vi "Capture the Project refs.vi"(8 "error in":errorcluster, 11 "Project Selection":string) -> (0 "error out":errorcluster, 3 "References":T1)   [LabVIEW 2019, in "Panther Dashboard.lvlib"]
uses:
  Panther Dashboard.lvlib
  Project References--cluster.ctl
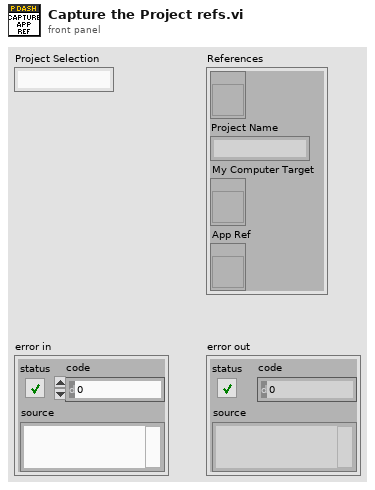
[diagram p1: front panel]
types:
  T1 = typedef "Panther Dashboard.lvlib/Project References--cluster.ctl" = cluster{"Project Ref":refnum<vi>, "Project Name":string, "My Computer Target":refnum<vi>, "App Ref":refnum<vi>}
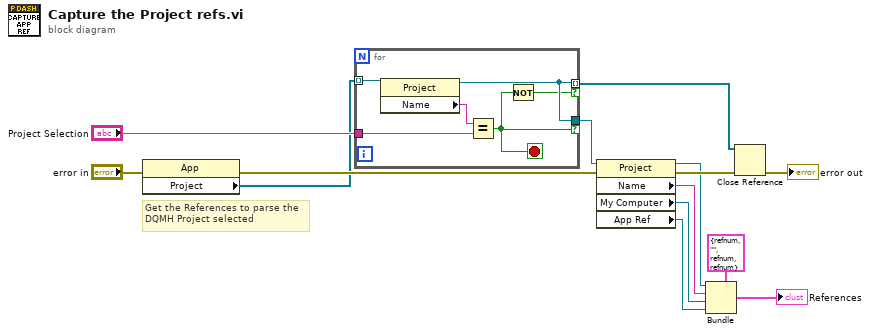
[diagram p0: block diagram]
diagram:
  # "Get the References to parse the\nDQMH Project selected"
  n1 = property class="App"(error in="error in") -> (error out=w13:errorcluster, "Project"=w2:refnum<vi>[])  [unwired: 1 in, 1 out]
  n2 = for {
    tunnel: w2 -> [w20] mode=indexing
    tunnel: [w17] -> w9 if=w16
    tunnel: "Project Selection" -> [w18]
    tunnel: [w17] -> w1 mode=indexing if=w15
    stop <- w16 stop-if-true
    n3 = property class="Project"(reference=w20) -> (reference out=w17:refnum<vi>, "Name"=w19:string)  [unwired: 1 in, 1 out]
    n4 = Equal?(x=w19, y=w18) -> (x = y?=w16:bool)
    n5 = Not(x=w16) -> (.not. x?=w15:bool)
  }
  n6 = property class="Project"(reference=w9, error in=w13) -> (reference out=w8:refnum<vi>, error out=w12:errorcluster, "Name"=w7:string, "My Computer"=w6:refnum<vi>, "App Ref"=w5:refnum<vi>)
  n7 = Bundle(cluster=T1 {"Project Ref"=refnum, "Project Name"="", "My Computer Target"=refnum, "App Ref"=refnum} ("References"), "Project Ref"=w8, "Project Name"=w7, "My Computer Target"=w6, "App Ref"=w5) -> (→"References":T1)
  n8 = Close Reference(reference=w1, error in (no error)=w12) -> (error out=→"error out":errorcluster)
